vi "PIM Panel.vi"(5 "PIM Driver Name/Configuration":string, 7 "PIM Command":T10, 8 "error in (no error)":errorcluster, 11 "Stimulus":T2={"Carrier Frequencies"={"C1 Freq, MHz"=0.0, "C2 Freq, MHz"=0.0}, "Carrier Powers"={"C1 Power,dBm"=0.0, "C2 Power, dBm"=0.0}, "Measurement Parameters"={"IM Order"=0, "Averaging"=1, "Direction"=0, "Enable ALC?"=FALSE, "Enable SingleIM?"=FALSE, "Display Units"=enum."dBm", "VA Hold?"=FALSE, "DUT PORT"=enum."Port 1"}, "Measurement Setup"={"Meas Type"=enum."Time", "TXStep"=0}} {"Measurement Setup"."TXStep" items=[".2", ".4", "1.0", "2.0"]; "Measurement Parameters"."Direction" items=["Reverse", "Forward", "Auxiliary"]; "Measurement Parameters"."IM Order" items=["3rd", "5th", "7th", "9th", "11th", "13th", "15th", "17th", "19th", "21st", "23rd", "25th", "27th", "29th", "31st", "33rd"]; "Measurement Parameters"."Averaging" items=["None", "Minimum", "Normal", "High", "Maximum"]}) -> (0 "error out":errorcluster, 2 "Variant Output":string, 3 "Measurement Results":T1 {"IMPower_dBc(s)" format="%.2f"; "TxFreqs" format="%.2f"; "IMFreq(s)" format="%.2f"; "IMPower(s)" format="%.2f"; "TxPower" format="%.2f"})   [LabVIEW 2011]
uses:
  PIM Command.ctl
  PIM Stimulus.ctl
  PIM Cmd Params.ctl
  SI.LIB/PIM.LIB/HW IO/IMOrder.ctl
  SI.LIB/PIM.LIB/HW IO/HW Averaging.ctl
  SI.LIB/PIM.LIB/HW IO/MeasMode.ctl
  SI.LIB/PIM.LIB/DISPLAY/display_unit_format.ctl
  SI.LIB/PIM.LIB/HW IO/DUTport.ctl
  SI.LIB/PIM.LIB/HW IO/PIM Sweep Step Size.ctl
  PIM Results.ctl
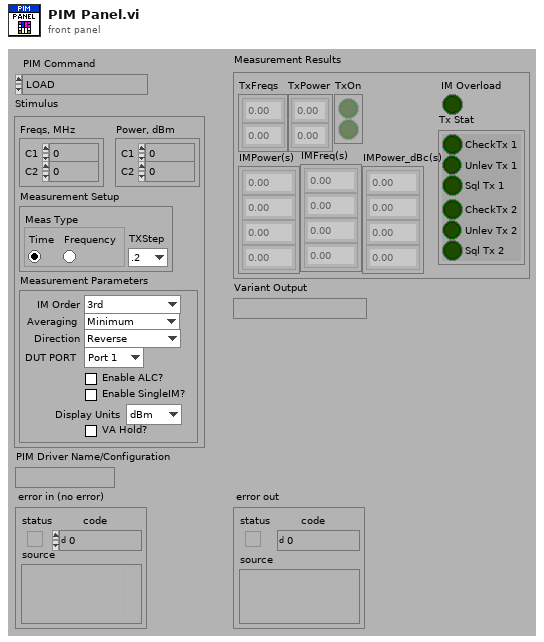
[diagram p1: front panel]
types:
  T1 = typedef "PIM Results.ctl" = cluster{"TxFreqs":dbl[], "TxPower":dbl[], "TxOn":bool[], "IMPower(s)":dbl[], "IMFreq(s)":dbl[], "Tx Stat":cluster{"CheckTx 1":bool, "Unlev Tx 1":bool, "Sql Tx 1":bool, "CheckTx 2":bool, "Unlev Tx 2":bool, "Sql Tx 2":bool}, "IM Overload":bool, "IMPower_dBc(s)":dbl[]}
  T2 = typedef "PIM Stimulus.ctl" = cluster{"Carrier Frequencies":cluster{"C1 Freq, MHz":dbl, "C2 Freq, MHz":dbl}, "Carrier Powers":cluster{"C1 Power,dBm":dbl, "C2 Power, dBm":dbl}, "Measurement Parameters":T3, "Measurement Setup":cluster{"Meas Type":enum32{"Time", "Frequency"}, "TXStep":T9}}
  T3 = typedef "PIM Cmd Params.ctl" = cluster{"IM Order":T4, "Averaging":T5, "Direction":T6, "Enable ALC?":bool, "Enable SingleIM?":bool, "Display Units":T7, "VA Hold?":bool, "DUT PORT":T8}
  T4 = typedef "IMOrder.ctl" = u8
  T5 = typedef "HW Averaging.ctl" = u16
  T6 = typedef "MeasMode.ctl" = u16
  T7 = typedef "display_unit_format.ctl" = enum16{"dBm", "dBc"}
  T8 = typedef "DUTport.ctl" = enum16{"Port 1", "Port 2"}
  T9 = typedef "PIM Sweep Step Size.ctl" = u16
  T10 = typedef "PIM Command.ctl" = enum16{"LOAD", "KEEP ALIVE", "VALIDATE", "INITIALIZE", "PRESET", "GET CALIBRATION", "SET STIMULUS", "TOGGLE TX POWER", "SET TX ON", "SET TX OFF", "MEASURE", "UNLOAD"}
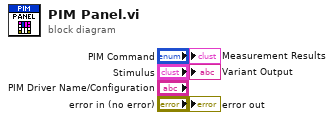
[diagram p0: block diagram]
diagram:
